vi "AlliGator Get-Set Phasor Ratio References.vi"(0 "Reference Phasor 1":T1, 1 "Reference Frequency 1":dbl[unit], 5 "Reference Lifetime 1":dbl[unit], 7 "Reference Phasor 2":T1, 9 "Reference Lifetime 2":dbl[unit], 11 "error in (no error)":errorcluster, 12 "Reference Frequency 2":dbl[unit], 13 "Get(F)/Set":bool) -> (2 "All defined?":bool, 3 "Reference Frequency 1":dbl[unit], 4 "Reference Phasor 1":T1, 6 "Reference Lifetime 1":dbl[unit], 8 "Reference Phasor 2":T1, 10 "Reference Lifetime 2":dbl[unit], 14 "Reference Frequency 2":dbl[unit], 15 "error out":errorcluster)   [LabVIEW 2021, in "AlliGator Phasor Ratio.lvlib"]
doc: "Stores the references and their associated data."
uses:
  Phasor/Phasor (g, s).ctl
  AlliGator Variables List.ctl
  AlliGator Phasor Ratio.lvlib
  AlliGator Globals, Variables & Constants.lvlib
  Phasor/Phasor.lvlib
panel:
  # "see the AlliGator License on the block diagram (Ctrl+E or Window:Show Block Diagram)"
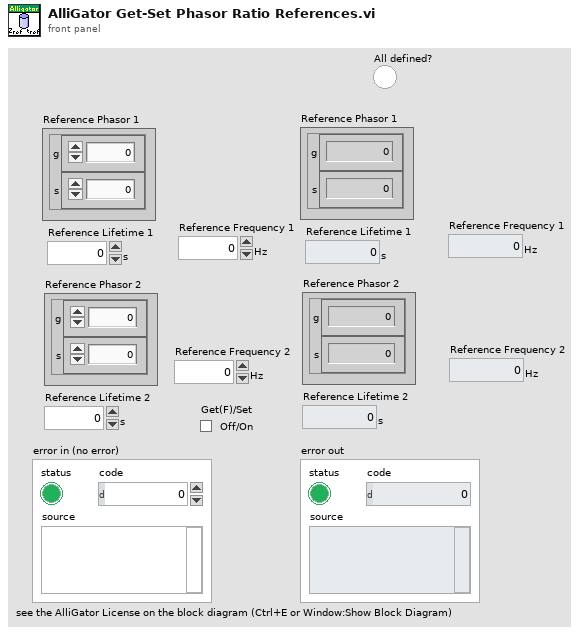
[diagram p1: front panel]
types:
  T1 = typedef "Phasor.lvlib/Phasor (g, s).ctl" = cluster{"g":dbl, "s":dbl}
  T2 = typedef "AlliGator Globals, Variables & Constants.lvlib/AlliGator Variables List.ctl" = enum16{"---- GUI ----", "Initialization Status", "State Indicators Refnum", "Original AlliGator Menu Items", "Current Action Loop State", "Script in progress", "Playback", "Loop Playback", "Search ROI Used", "Search ROI", "Decay Graph Max Legend Size", "Intensity Graph Max Legend Size", "Decay Statistics Graph Max Legend Size", "Phasor Graph Max Legend Size", "Phasor Ratio Graph Max Legend Size", "Lifetime Graph Max Legend Size", "---- Files ----", "Export Dataset Frames as Individual Files", "Show Batch Export Help Balloons", "Frames in Dataset", "ptu File Frame Start Indices", "Current Frame in Dataset", "Current Frame Timestamp", "------ Python Plugins ------", "Python Plugins Information", "Python Session", "Valid Python Session?", "---- Source Image ----", "Dataset Loaded", "Dataset Metadata", "Dataset Channel", "Dataset Data Description", "Background Dataset Metadata", "Background Dataset Channel", "Background Dataset Data Description", "Background File Subtraction", "Background File Path", "Background File Pile-up Correction", "Background File Pixel Well Capacity", "Background File Scaling Factor", "Source Image ROIs", "Current Source Image ROI", "Source Image ROI Event Refnum", "X_Source Image Display Range", "X_Source Image Palette Information", "Source Image Palette List", "Source Image Scale", "Current Dataset Load Settings", "Source Image:ROI Overlay Color", "---- Image Profile Window ----", "Image Profile:Overlay ROI in Source Image", "Image Profile Window Event Refnum", "Image Profile:IntensityType", "Image Profile:Intensity Average Type", "Image Profile:Intensity-weighted SDV", "Image Profile:Box Profile Type", "Image Profile Window Open", "Image Profile:Plotted Fit Parameter", "X_Type of Displayed Image", "X_Time Gate Slider", "Dataset Path", "Source Image Overlay to Erase", "Is Displayed Image Accumulated", "White Light Image Modified", "Mask Image Modified", "Macrotime Gate Separation", "------ Phasor Graph -------", "Phasor Graph:Show Line", "---- Phasor Plot ---", "Phasor Plot Parameters Changed", "FLI Dataset Modified since last Phasor Plot Calculation", "Phasor Harmonics Data", "Selected Phasor Harmonics", "Phasor Harmonic Manager Event Refnum", "Phasor Plot ROIs", "Current Phasor Plot ROI", "Phasor Plot ROI Event Refnum", "Phasor Plot Image Reference Points", "Phasor Plot Computed", "Phasor Plot Palette Information", "Phasor Plot Palette List", "Phasor Ratio Palette Information", "Phasor Ratio Palette List", "Phasor Image Scale", "Phasor Plot Image Overlay to Erase", "Phasor Plot Image Elements to Update", "Current Phasor Plot Calculation Parameters", "Current Phasor Calibration Options", "Reset Cumulated Phasor Plot", "Phasor Ratio Reference 1", "Phasor Ratio Lifetime Reference 1", "Phasor Ratio Reference 1 Frequency", "Phasor Ratio Reference 2", "Phasor Ratio Lifetime Reference 2", "Phasor Ratio Reference 2 Frequency", "---- Decay Analysis ----", "Number of Selected Decays to Fit", "LS Fit Results", "LAR Fit Results", "BS Fit Results", "Last Decay Max - Min", "Best Fit Parameters", "Best Fit Parameter Names", "Actual Size X", "Actual Size Y", "Binning X", "Binning Y", "Actual # Gates", "Dataset Number", "Gates to...", "Gates Skipped", "Gates to keep", "Gate Step", "Gate Separation", "Reversed Gates", "Pile-up Correction", "Pixel Well Capacity", "Background Subtracted", "Background Subtraction Method", "Background Definition Range", "Background File (deprecated)", "Number of Dataset Accumulated", "Array of Accumulated Dataset Paths", "Do Averaged Datasets", "Destination File Path", "Process Plot Target", "Use 1/D as Phasor Frequency", "---- Decay Fit Parameter Map -----", "Decay Fit Parameter Map Palette Information", "Decay Fit Parameter Map Palette List", "Local Decay Graph Window Event Refnum", "------- Local Decay Window ---------", "Use normalized IRF for convolution", "----- Miscellaneous ----", "Skippable Dialog Windows Status"}
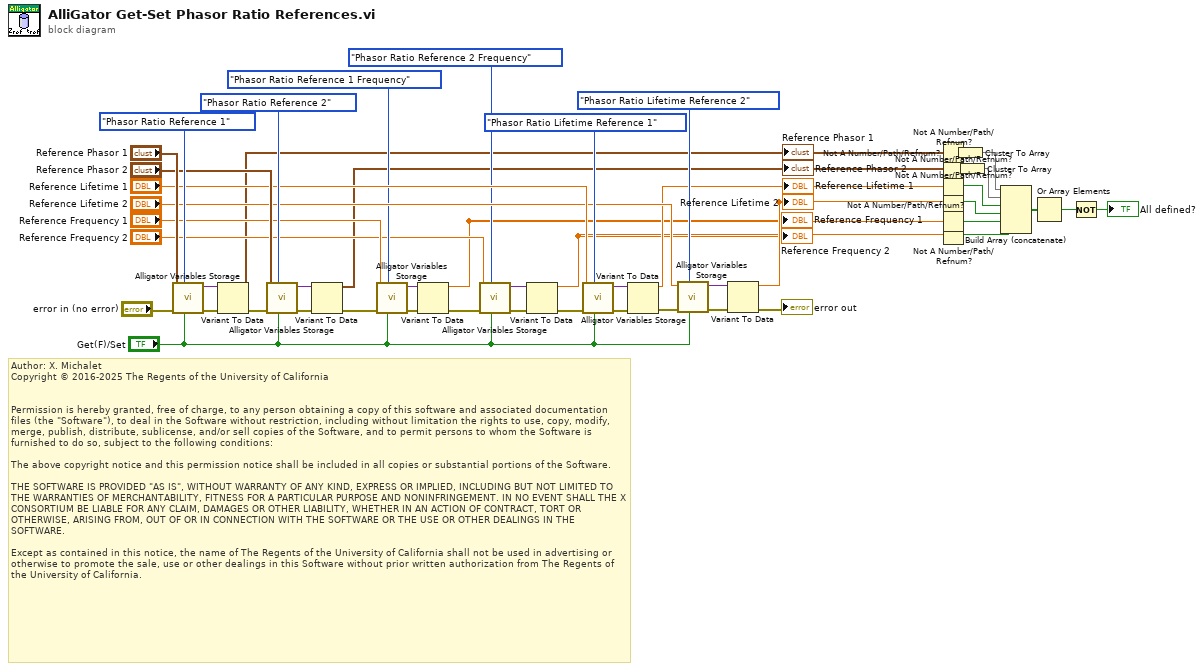
[diagram p0: block diagram]
diagram:
  # "Author: X. Michalet\nCopyright © 2016-2025 The Regents of the University of California\n \n\nPermission is hereby granted, free of charge, to any person obtaining a copy of this software and associated documentation files (the \"Software\"), to deal in the Software without restriction, including without limitation the rights to use, copy, modify, merge, publish, distribute, sublicense, and/or sell copies of the Software, and to permit persons to whom the Software is furnished to do so, subject to the following conditions:\n\nThe above copyright notice and this permission notice shall be included in all copies or substantial portions of the Software.\n\nTHE SOFTWARE IS PROVIDED \"AS IS\", WITHOUT WARRANTY OF ANY KIND, EXPRESS OR IMPLIED, INCLUDING BUT NOT LIMITED TO THE WARRANTIES OF MERCHANTABILITY, FITNESS FOR A PARTICULAR PURPOSE AND NONINFRINGEMENT. IN NO EVENT SHALL THE X CONSORTIUM BE LIABLE FOR ANY CLAIM, DAMAGES OR OTHER LIABILITY, WHETHER IN AN ACTION OF CONTRACT, TORT OR OTHERWISE, ARISING FROM, OUT OF OR IN CONNECTION WITH THE SOFTWARE OR THE USE OR OTHER DEALINGS IN THE SOFTWARE.\n\nExcept as contained in this notice, the name of The Regents of the University of California shall not be used in advertising or otherwise to promote the sale, use or other dealings in this Software without prior written authorization from The Regents of the University of California."
  n1 = call "Alligator Variables Storage.vi"("Get(F)/Set"="Get(F)/Set", "AlliGator Variable"=AlliGator_Variables_List."Phasor Ratio Reference 1" ("Alligator Variable"), "Error In"="error in (no error)", "Data in"="Reference Phasor 1") -> ("Error Out"=w42:errorcluster, "Data out"=w44:variant)  [unwired: 5 in, 1 out]
  n2 = Variant To Data(error in=w42, Variant=w44) -> (data=w17:T1, error out=w45:errorcluster)  [unwired: 1 in]
  "Reference Phasor 1" <- w17
  n3 = call "Alligator Variables Storage.vi"("Get(F)/Set"="Get(F)/Set", "AlliGator Variable"=AlliGator_Variables_List."Phasor Ratio Reference 2" ("Alligator Variable"), "Error In"=w45, "Data in"="Reference Phasor 2") -> ("Error Out"=w47:errorcluster, "Data out"=w41:variant)  [unwired: 5 in, 1 out]
  n4 = Variant To Data(error in=w47, Variant=w41) -> (data=w16:T1, error out=w29:errorcluster)  [unwired: 1 in]
  "Reference Phasor 2" <- w16
  n5 = call "Alligator Variables Storage.vi"("Get(F)/Set"="Get(F)/Set", "AlliGator Variable"=AlliGator_Variables_List."Phasor Ratio Reference 1 Frequency" ("Alligator Variable"), "Error In"=w29, "Data in"="Reference Frequency 1") -> ("Error Out"=w27:errorcluster, "Data out"=w26:variant)  [unwired: 5 in, 1 out]
  n6 = Variant To Data(error in=w27, Variant=w26) -> (data=w13:dbl[unit], error out=w25:errorcluster)  [unwired: 1 in]
  "Reference Frequency 1" <- w13
  n7 = call "Alligator Variables Storage.vi"("Get(F)/Set"="Get(F)/Set", "AlliGator Variable"=AlliGator_Variables_List."Phasor Ratio Reference 2 Frequency" ("Alligator Variable"), "Error In"=w25, "Data in"="Reference Frequency 2") -> ("Error Out"=w24:errorcluster, "Data out"=w22:variant)  [unwired: 5 in, 1 out]
  n8 = Variant To Data(error in=w24, Variant=w22) -> (data=w12:dbl[unit], error out=w23:errorcluster)  [unwired: 1 in]
  "Reference Frequency 2" <- w12
  n9 = call "Alligator Variables Storage.vi"("Get(F)/Set"="Get(F)/Set", "AlliGator Variable"=AlliGator_Variables_List."Phasor Ratio Lifetime Reference 1" ("Alligator Variable"), "Error In"=w23, "Data in"="Reference Lifetime 1") -> ("Error Out"=w35:errorcluster, "Data out"=w36:variant)  [unwired: 5 in, 1 out]
  n10 = Variant To Data(error in=w35, Variant=w36) -> (data=w15:dbl[unit], error out=w37:errorcluster)  [unwired: 1 in]
  "Reference Lifetime 1" <- w15
  n11 = call "Alligator Variables Storage.vi"("Get(F)/Set"="Get(F)/Set", "AlliGator Variable"=AlliGator_Variables_List."Phasor Ratio Lifetime Reference 2" ("Alligator Variable"), "Error In"=w37, "Data in"="Reference Lifetime 2") -> ("Error Out"=w38:errorcluster, "Data out"=w39:variant)  [unwired: 5 in, 1 out]
  n12 = Variant To Data(error in=w38, Variant=w39) -> (data=w14:dbl[unit], error out=→"error out":errorcluster)  [unwired: 1 in]
  "Reference Lifetime 2" <- w14
  n13 = Not A Number/Path/Refnum?(number/path/refnum=w17) -> (NaN/Path/Refnum?=w6:cluster{"g":bool, "s":bool})
  n14 = Not A Number/Path/Refnum?(number/path/refnum=w16) -> (NaN/Path/Refnum?=w7:cluster{"g":bool, "s":bool})
  n15 = Not A Number/Path/Refnum?(number/path/refnum=w15) -> (NaN/Path/Refnum?=w8:bool)
  n16 = Not A Number/Path/Refnum?(number/path/refnum=w14) -> (NaN/Path/Refnum?=w9:bool)
  n17 = Not A Number/Path/Refnum?(number/path/refnum=w13) -> (NaN/Path/Refnum?=w10:bool)
  n18 = Not A Number/Path/Refnum?(number/path/refnum=w12) -> (NaN/Path/Refnum?=w11:bool)
  n19 = Cluster To Array(cluster=w6) -> (array=w4:bool[])
  n20 = Cluster To Array(cluster=w7) -> (array=w5:bool[])
  n21 = Build Array (concatenate)(w4, w5, w8, w9, w10, w11) -> (w3:bool[])
  n22 = Or Array Elements(Boolean array=w3) -> (logical OR=w2:bool)
  n23 = Not(x=w2) -> (.not. x?=→"All defined?":bool)
